vi "Acquisition Engine Pre-Trigger Storage (FIFO).vi"(5 "FIFO Out":refnum<k21>="HistoryFIFOU128", 6 "states":T1, 8 "Trigger Info":cluster{"Trigger":bool, "Trig Offset":u8}, 9 "PostTrigComplete":bool, 10 "AcqInProgress":bool, 11 "Input Data":i16[](array[numeric])=[0, 0, 0, 0, 0, 0, 0, 0]) -> (0 "Trigger Info":cluster{"Trigger":bool, "Trig Offset":u8}, 1 "Output Valid":bool, 3 "Output Data":i16[](array[numeric]), 7 "Flushed":bool)   [LabVIEW 2012]
uses:
  <instrlib>/FlexRIO/Libraries/Acquisition Engine/FPGA/Interface/acqEngineStates v1.ctl
  <vilib>/rvi/FXPMathLib/basic elements/FxpDiscreteDelay/XNode/nifxpmath_DiscreteDelay.xnode
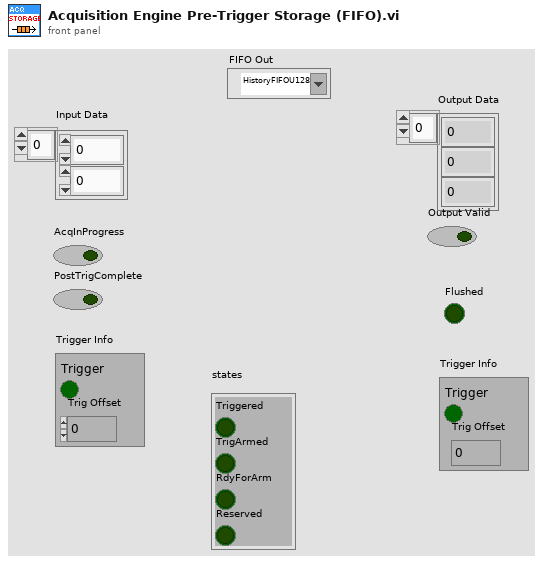
[diagram p1: front panel]
types:
  T1 = typedef "acqEngineStates v1.ctl" = cluster{"Triggered":bool, "TrigArmed":bool, "RdyForArm":bool, "Reserved":bool}
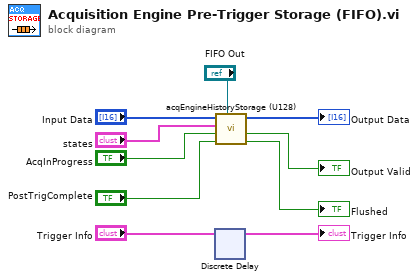
[diagram p0: block diagram]
diagram:
  n1 = xnode "Discrete Delay"("D"="Trigger Info") -> ("Q"=→"Trigger Info":cluster{"Trigger":bool, "Trig Offset":u8})
  n2 = call <userlib>:"acqEngineHistoryStorage (U128).vi"("FIFO Out"="FIFO Out", "PostTrigComplete"="PostTrigComplete", "AcqInProgress"="AcqInProgress", "states"="states", "Input Data"="Input Data") -> ("flushed"=→"Flushed":bool, "valid"=→"Output Valid":bool, "Output Data"=→"Output Data":i16[])  [unwired: 4 in]
